vi "HMI-Reactor.vi"() -> ()   [LabVIEW 2017]
panel:
  out "CA":dbl=456.3558684423593 format="%#_3g"
  out "CA0":dbl=2000.0 format="%#_3g"
  out "10SDV502":bool=TRUE
  out "?":dbl format="%#_3g"
  in  "10HIC300":dbl=50.0
  out "TJ":dbl=365.3749789937039 format="%#_3g"
  out "T":dbl=333.97788169438996 format="%#_3g"
  out "Reactor Temp":T1={"% Opening"=0.0, "SP"=0.0, "Reactor Temp"=333.97788169438996, "Temp"=333.97788169438996} {"Temp" format="%#_4g"; "Reactor Temp" scale=0.0..700.0; "SP" scale=0.0..700.0; "% Opening" scale=0.0..100.0}
  in  "10TIC100 Faceplate":T2={"PID Parameters"={"KP"=1.0, "KI"=0.01, "KD"=0.0}, "M"=FALSE, "SP_VAL"=0.0, "% Open"=50.0}
  out "?":dbl format="%#_3g"
  out "10SDV501":bool=TRUE
  out "FJ":dbl=15.0 format="%#_3g"
  out "TJ0":dbl=300.0 format="%#_3g"
  out "10SDV500":bool=TRUE
  out "F0":dbl=1.0 format="%#_3g"
  out "T0":dbl=323.0 format="%#_3g"
  out "Reactor Level":T3={"% Opening"=0.0, "SP"=0.0, "Reactor Level"=54.508701366151044, "Level"=54.508701366151044} {"Level" format="%#_4g"; "Reactor Level" scale=0.0..100.0; "SP" scale=0.0..100.0; "% Opening" scale=0.0..100.0}
  out "?":dbl format="%#_3g"
  in  "10LIC200 Faceplate":T2={"PID Parameters"={"KP"=1.0, "KI"=0.01, "KD"=0.0}, "M"=FALSE, "SP_VAL"=0.0, "% Open"=50.0}
  out "10-R-100":dbl(slide)=54.508701366151044 scale=0.0..100.0 scale format="%#_4g"
  in  "stop":bool
  # "m3/min"
  # "Mole/m3"
  # "10LV200"
  # "%"
  # "K"
  # "%"
  # "K"
  # "m3/min"
  # "10TV100"
  # "%"
  # "K"
  # "Mole/m3"
  # "%"
  # "K"
  # "A"
  # "%"
  # "A"
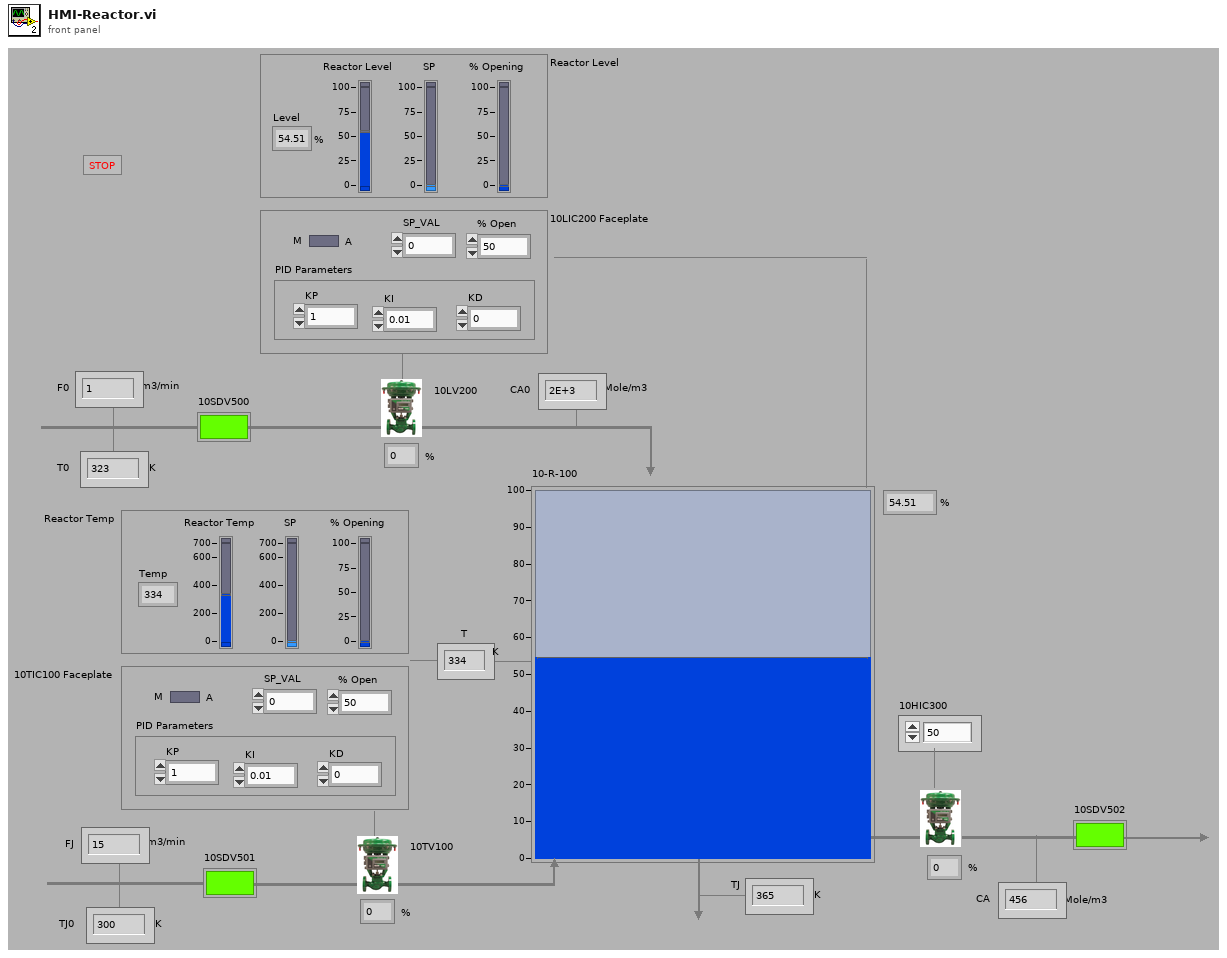
[diagram p1: front panel]
types:
  T1 = cluster{"% Opening":dbl, "SP":dbl, "Reactor Temp":dbl, "Temp":dbl}
  T2 = cluster{"PID Parameters":cluster{"KP":dbl, "KI":dbl, "KD":dbl}, "M":bool, "SP_VAL":dbl, "% Open":dbl}
  T3 = cluster{"% Opening":dbl, "SP":dbl, "Reactor Level":dbl, "Level":dbl}
  T4 = cluster{"% Open":dbl, "SP_VAL":dbl, "Double":dbl, "Double":dbl}
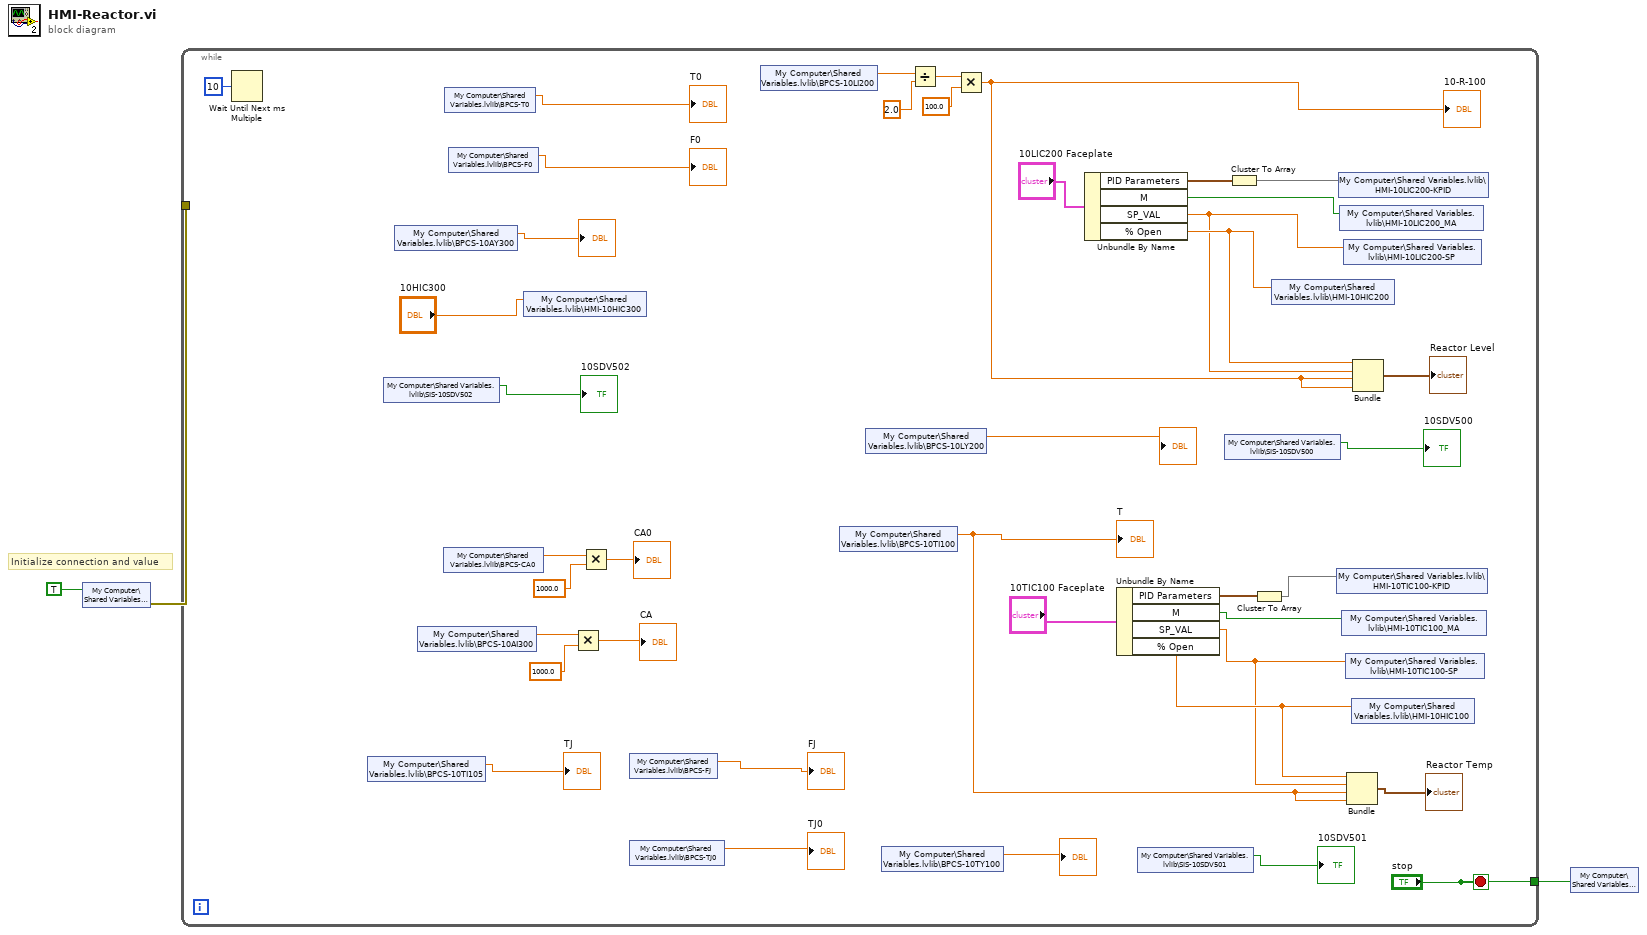
[diagram p0: block diagram]
diagram:
  # "Initialize connection and value"
  n1 = shared-variable "My Computer\\Shared Variables.lvlib\\stop"(TRUE) -> (error out=w2:errorcluster)  [unwired: 1 in]
  n2 = while {
    tunnel: ["stop"] -> w3
    tunnel: w2 -> [_]
    stop <- "stop" stop-if-true
    n3 = Wait Until Next ms Multiple(millisecond multiple=u32 10) -> ()  [unwired: 1 out]
    n4 = shared-variable "My Computer\\Shared Variables.lvlib\\BPCS-10TI105"() -> (→"TJ":dbl)  [unwired: 1 in, 1 out]
    n5 = shared-variable "My Computer\\Shared Variables.lvlib\\SIS-10SDV502"() -> (→"10SDV502":bool)  [unwired: 1 in, 1 out]
    n6 = shared-variable "My Computer\\Shared Variables.lvlib\\BPCS-10AY300"() -> (→"?":dbl)  [unwired: 1 in, 1 out]
    n7 = shared-variable "My Computer\\Shared Variables.lvlib\\BPCS-10AI300"() -> (w9:dbl)  [unwired: 1 in, 1 out]
    n8 = shared-variable "My Computer\\Shared Variables.lvlib\\BPCS-CA0"() -> (w12:dbl)  [unwired: 1 in, 1 out]
    n9 = shared-variable "My Computer\\Shared Variables.lvlib\\BPCS-T0"() -> (→"T0":dbl)  [unwired: 1 in, 1 out]
    n10 = shared-variable "My Computer\\Shared Variables.lvlib\\BPCS-F0"() -> (→"F0":dbl)  [unwired: 1 in, 1 out]
    n11 = shared-variable "My Computer\\Shared Variables.lvlib\\HMI-10HIC300"("10HIC300") -> ()  [unwired: 1 in, 1 out]
    n12 = Multiply(x=w9, y=1000.0) -> (x*y=→"CA":dbl)
    n13 = Multiply(x=w12, y=1000.0) -> (x*y=→"CA0":dbl)
    n14 = shared-variable "My Computer\\Shared Variables.lvlib\\BPCS-FJ"() -> (→"FJ":dbl)  [unwired: 1 in, 1 out]
    n15 = shared-variable "My Computer\\Shared Variables.lvlib\\BPCS-TJ0"() -> (→"TJ0":dbl)  [unwired: 1 in, 1 out]
    n16 = shared-variable "My Computer\\Shared Variables.lvlib\\BPCS-10LI200"() -> (w5:dbl)  [unwired: 1 in, 1 out]
    n17 = shared-variable "My Computer\\Shared Variables.lvlib\\BPCS-10TI100"() -> (w23:dbl)  [unwired: 1 in, 1 out]
    "T" <- w23
    n18 = shared-variable "My Computer\\Shared Variables.lvlib\\BPCS-10LY200"() -> (→"?":dbl)  [unwired: 1 in, 1 out]
    n19 = shared-variable "My Computer\\Shared Variables.lvlib\\BPCS-10TY100"() -> (→"?":dbl)  [unwired: 1 in, 1 out]
    n20 = Divide(x=w5, y=2.0 ("x")) -> (x/y=w40:dbl)
    n21 = Multiply(x=w40, y=100.0) -> (x*y=w4:dbl)
    "10-R-100" <- w4
    n22 = Unbundle By Name("10LIC200 Faceplate") -> ("PID Parameters"=w37:cluster{"KP":dbl, "KI":dbl, "KD":dbl}, "M"=w35:bool, "SP_VAL"=w33:dbl, "% Open"=w34:dbl)
    n23 = Unbundle By Name("10TIC100 Faceplate") -> ("PID Parameters"=w29:cluster{"KP":dbl, "KI":dbl, "KD":dbl}, "M"=w27:bool, "SP_VAL"=w25:dbl, "% Open"=w26:dbl)
    n24 = shared-variable "My Computer\\Shared Variables.lvlib\\SIS-10SDV501"() -> (→"10SDV501":bool)  [unwired: 1 in, 1 out]
    n25 = shared-variable "My Computer\\Shared Variables.lvlib\\SIS-10SDV500"() -> (→"10SDV500":bool)  [unwired: 1 in, 1 out]
    n26 = Cluster To Array(cluster=w37) -> (array=w36:dbl[])
    n27 = Cluster To Array(cluster=w29) -> (array=w28:dbl[])
    n28 = shared-variable "My Computer\\Shared Variables.lvlib\\HMI-10HIC200"(w34) -> ()  [unwired: 1 in, 1 out]
    n29 = shared-variable "My Computer\\Shared Variables.lvlib\\HMI-10TIC100-KPID"(w28) -> ()  [unwired: 1 in, 1 out]
    n30 = shared-variable "My Computer\\Shared Variables.lvlib\\HMI-10LIC200-KPID"(w36) -> ()  [unwired: 1 in, 1 out]
    n31 = shared-variable "My Computer\\Shared Variables.lvlib\\HMI-10LIC200_MA"(w35) -> ()  [unwired: 1 in, 1 out]
    n32 = shared-variable "My Computer\\Shared Variables.lvlib\\HMI-10TIC100_MA"(w27) -> ()  [unwired: 1 in, 1 out]
    n33 = shared-variable "My Computer\\Shared Variables.lvlib\\HMI-10LIC200-SP"(w33) -> ()  [unwired: 1 in, 1 out]
    n34 = shared-variable "My Computer\\Shared Variables.lvlib\\HMI-10TIC100-SP"(w25) -> ()  [unwired: 1 in, 1 out]
    n35 = Bundle("% Open"=w26, "SP_VAL"=w25, "Double"=w23, "Double"=w23) -> (→"Reactor Temp":T4)  [unwired: 1 in]
    n36 = shared-variable "My Computer\\Shared Variables.lvlib\\HMI-10HIC100"(w26) -> ()  [unwired: 1 in, 1 out]
    n37 = Bundle("% Open"=w34, "SP_VAL"=w33, w4, w4) -> (→"Reactor Level":cluster{"% Open":dbl, "SP_VAL":dbl, dbl, dbl})  [unwired: 1 in]
  }
  n38 = shared-variable "My Computer\\Shared Variables.lvlib\\stop"(w3) -> ()  [unwired: 1 in, 1 out]
